vi "NanotecSMCPD.ProcPeriodic.vi"(0 "i ref in":refnum<vi>, 3 "ms timeout (10000)":i32=10000, 5 "error in (no error)":errorcluster) -> (14 "i ref out":refnum<vi>, 17 "timed out":bool, 19 "error out":errorcluster)   [LabVIEW 2014, in "NanotecSMCPD.lvlib"]
doc: "This method serves to periodically do things like reading values from the HW. Methods that should be executed periodically should be called from THIS method. Add code here."
uses:
  NanotecSMCPD.lvlib
  CSCore/CSSystem/CoreDefs/CoreDefs.error_type.ctl
  CSCore/CSSystem/CoreDefs/CoreDefs.error_severity.ctl
  CSCore/CSApplicationBaseClasses/MotorBase/MotorBase.statusType.ctl
  CSCore/CSApplicationBaseClasses/MotorBase/MotorBase.lvlib
  CSCore/CSSystem/CoreLib/CoreLib.lvlib
  CSlibraries/UtilityLib/UtilityLib.lvlib
  CSlibraries-extern/DimLVEvent/LVDimInterface/LVDimInterface.lvlib
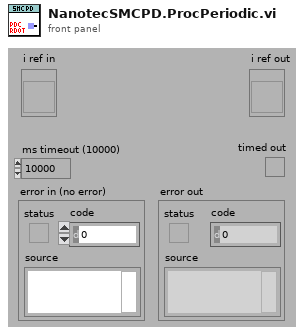
[diagram p1: front panel]
types:
  T1 = typedef "CoreDefs.error_severity.ctl" = enum16{"undefined", "information", "warning", "error", "fatal"}
  T2 = typedef "CoreDefs.error_type.ctl" = enum16{"no error", "can't load process", "can't unload process", "process does not exist", "can't install process", "can't remove process", "unknown function", "time out", "can't execute function", "duplicate queue name", "super not found", "caller queue invalid", "can't ping process", "unknown error", "VISA Error", "VISA timeout", "GPIB timeout", "GPIB error", "communication error", "data type mismatch", "can't read data from OPC server", "can't write data to OPC server", "OET error", "function not implemented", "process already exists", "invalid Shared Variable name", "error writing Shared Variable", "error reading Shared Variable", "invalid client name", "corrupt database", "unknown class", "call not authorized", "parameter out of range", "OET timeout: can't get data to modify", "invalid queue name", "requested operation incompatible with current state", "event undefined", "event disabled", "state undefined", "caller is not a friend", "EventBuilder: bad eventID", "EventBuilder: no DAQ devices", "a thread must not stop itself", "UNUSED ELEMENT4", "DiscArchiver: eventData incomplete", "DiscArchiver: eventData does not belong to run", "DiscArchiver: can't open file", "DiscArchiver: can't write to file", "DiscArchiver: available disc space low", "can't acquire semaphore", "error reading data from database", "notifier object is not existing", "can't register process", "can't unregister process", "illegal event type", "object disabled", "object already exists", "can't change state", "Instrument not found", "no connection to remote node", "invalid reference", "N/A", "UNUSED ELEMENT 1", "element not found", "illegal TCP/IP connection detected", "object does not exist", "invalid access ID", "unknown CS system", "invalid privilige", "unsupported data type", "unsupported server type", "IO server already exists", "Shared Variable already exists"}
  T3 = typedef "MotorBase.lvlib/MotorBase.statusType.ctl" = u32
  T4 = typedef "NanotecSMCPD.lvlib/NanotecSMCPD.i attribute.ctl" = cluster{"referencing":bool[], "stop":bool[], "AutoHalt ID":i32, "MethodQueue":refnum<queue>, "Referenced1Time?":bool[], "LastCommand ID":i32}
  T5 = cluster{"Method":enum16{"MoveRelative", "MoveAbsolute", "Stop"}, "Axis":i32, "Steps":dbl}
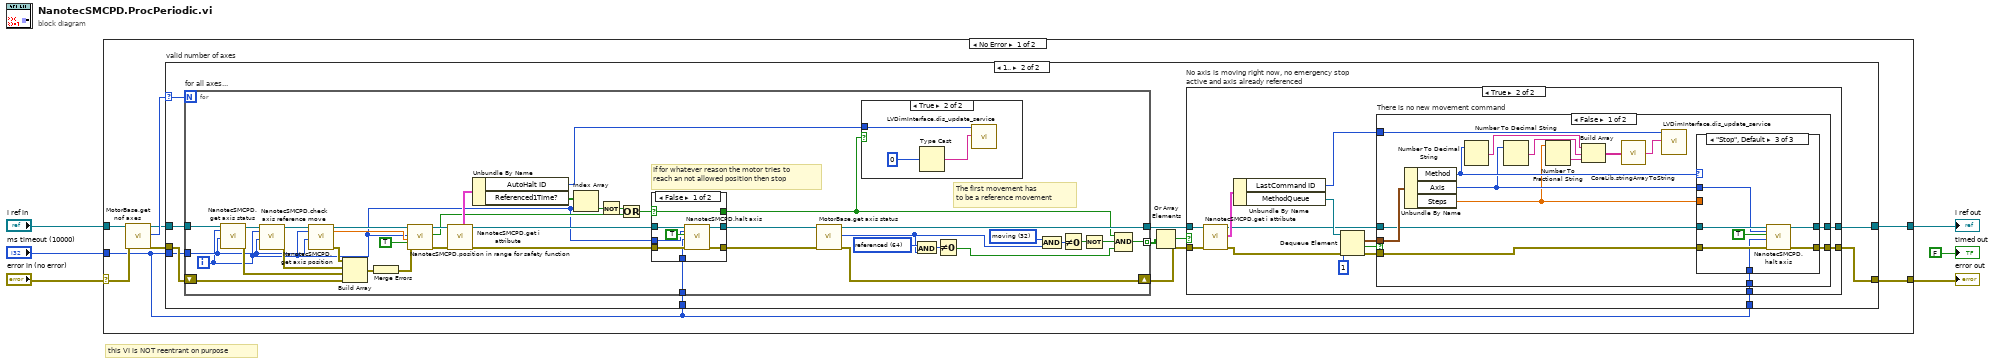
[diagram p0: block diagram]
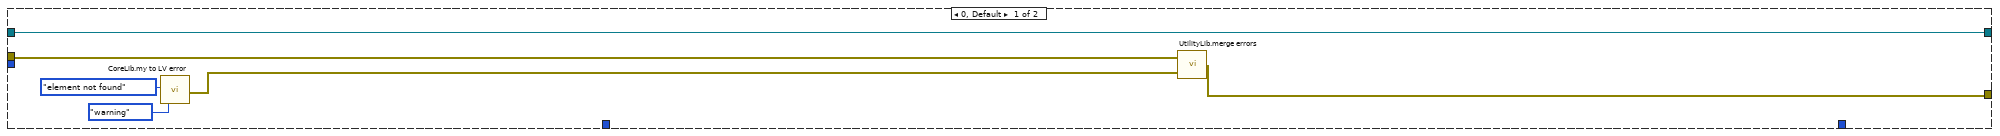
[diagram p2: hidden frame]
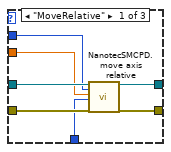
[diagram p4: hidden frame]
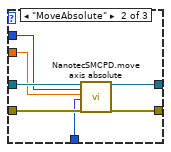
[diagram p5: hidden frame]
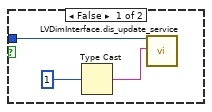
[diagram p7: hidden frame]
diagram:
  # "this VI is NOT reentrant on purpose"
  n1 = case shown="No Error" "error in (no error)" {
    selector: "error in (no error)" -> [w11 w144]
    tunnel: "i ref in" -> [w12 w145]
    tunnel: [w14 w145] -> w4
    tunnel: [w13 w144] -> w3
    tunnel: "ms timeout (10000)" -> [w7 _]
    frame No Error {
      n2 = call "MotorBase.get nof axes.vi"("i ref in"=w12, "error in (no error)"=w11) -> ("i ref out"=w9:refnum<vi>, "nOfAxis"=w10:i32, "error out"=w8:errorcluster)  [unwired: 15 in]
      n3 = case "valid number of axes" shown="1.." w10 {
        selector: w10 -> [_ w30]
        tunnel: [w20 w24] -> w14
        tunnel: w9 -> [w20 w32]
        tunnel: w8 -> [w17 w31]
        tunnel: [w15 w23] -> w13
        tunnel: w7 -> [_ w29]
        tunnel: w7 -> [_ w25]
        tunnel: w7 -> [_ w21]
        frame 0, Default {
          n4 = call "CoreLib.my to LV error.vi"("ErrorTypes"=CoreDefs.error_type."element not found", "severityLevel"=CoreDefs.error_severity."warning") -> ("myErrorCluster"=w16:errorcluster)  [unwired: 16 in, 1 out]
          n5 = call "UtilityLib.merge errors.vi"("error2 (no error)"=w16, "error1 (no error)"=w17) -> ("error out"=w15:errorcluster)
        }
        frame 1.. {
          n6 = for "for all axes..." {
            N: w30 -> [_]
            tunnel: w32 -> [w87]
            shift-right: [w121] -> w26
            shift-left: w31 -> [w125]
            tunnel: w29 -> [w89]
            tunnel: [w120] -> w27
            tunnel: [w98] -> w28 mode=indexing
            tunnel: w21 -> [w104]
            i -> [w88]
            w116 = T3 64 items=["motorEnabled"=1, "negativeLimitSwitchActive"=2, "positiveLimitSwitchActive"=4, "limitSwitchesEnabled"=8, "limitSwitchesAreNormallyClosed"=16, "moving"=32, "referenced"=64, "inPosition"=128, "reserved2"=256, "reserved3"=512, "reserved4"=1024, "reserved5"=2048, "error"=4096, "reserved6"=8192, "reserved7"=16384, "reserved8"=32768, "user defined1"=65536, "user defined2"=131072, "user defined3"=262144, "user defined4"=524288, "user defined5"=1048576, "user defined6"=2097152, "user defined7"=4194304, "user defined8"=8388608, "user defined9"=16777216, "user defined10"=33554432, "user defined11"=67108864, "user defined12"=134217728, "user defined13"=268435456, "user defined14"=536870912, "user defined15"=1073741824, "user defined16"=2147483648] ("status")
            w122 = T3 32 items=["motorEnabled"=1, "negativeLimitSwitchActive"=2, "positiveLimitSwitchActive"=4, "limitSwitchesEnabled"=8, "limitSwitchesAreNormallyClosed"=16, "moving"=32, "referenced"=64, "inPosition"=128, "reserved2"=256, "reserved3"=512, "reserved4"=1024, "reserved5"=2048, "error"=4096, "reserved6"=8192, "reserved7"=16384, "reserved8"=32768, "user defined1"=65536, "user defined2"=131072, "user defined3"=262144, "user defined4"=524288, "user defined5"=1048576, "user defined6"=2097152, "user defined7"=4194304, "user defined8"=8388608, "user defined9"=16777216, "user defined10"=33554432, "user defined11"=67108864, "user defined12"=134217728, "user defined13"=268435456, "user defined14"=536870912, "user defined15"=1073741824, "user defined16"=2147483648] ("status")
            # "The first movement has\nto be a reference movement"
            # "If for whatever reason the motor tries to\nreach an not allowed position then stop"
            n7 = call "NanotecSMCPD.get axis status.vi"("i ref in"=w87, "axis"=w88, "ms timeout (10000)"=w89) -> ("i ref out"=w126:refnum<vi>, "error out"=w92:errorcluster)  [unwired: 12 in, 3 out]
            n8 = call "NanotecSMCPD.check axis reference move.vi"("i ref in"=w126, "axis"=w88, "ms timeout (10000)"=w89) -> ("i ref out"=w95:refnum<vi>, "error out"=w91:errorcluster)  [unwired: 14 in, 1 out]
            n9 = call "NanotecSMCPD.get axis position.vi"("i ref in"=w95, "axis"=w88, "ms timeout (10000)"=w89) -> ("i ref out"=w94:refnum<vi>, "position [unit]"=w93:dbl, "error out"=w90:errorcluster)  [unwired: 13 in, 1 out]
            n10 = Build Array(w90, w91, w92, w125) -> (w124:errorcluster[])
            n11 = Merge Errors(w124) -> (w119:errorcluster)
            n12 = call "NanotecSMCPD.position in range for safety function.vi"("i ref in"=w94, "axisIndex"=w88, "reqPosition"=w93, "absolute"=TRUE, "error in (no error)"=w119) -> ("i ref out"=w114:refnum<vi>, "in range"=w110:bool, "error out"=w113:errorcluster)  [unwired: 12 in]
            n13 = call "NanotecSMCPD.get i attribute.vi"("i ref in"=w114, "error in (no error)"=w113) -> ("i ref out"=w108:refnum<vi>, "i attribute"=w112:T4, "error out"=w107:errorcluster)  [unwired: 15 in]
            n14 = Unbundle By Name(w112) -> ("AutoHalt ID"=w96:i32, "Referenced1Time?"=w111:bool[])
            n15 = Index Array(array=w111, index=w88) -> (element=w103:bool)
            n16 = Not(x=w103) -> (.not. x?=w102:bool)
            n17 = Or(x=w102, y=w110) -> (x .or. y?=w109:bool)
            n18 = case shown="False" w109 {
              selector: w109 -> [w133 w141]
              tunnel: w108 -> [w139 w143]
              tunnel: w107 -> [w138 w142]
              tunnel: [w137 w143] -> w106
              tunnel: [w136 w142] -> w105
              tunnel: w88 -> [w135 _]
              tunnel: w104 -> [w134 _]
              tunnel: [w133 w141] -> w97
              frame False {
                n19 = call "NanotecSMCPD.halt axis.vi"("i ref in"=w139, "axis"=w135, "ManuelStop"=TRUE, "ms timeout (10000)"=w134, "error in (no error)"=w138) -> ("i ref out"=w137:refnum<vi>, "error out"=w136:errorcluster)  [unwired: 12 in, 1 out]
              }
              frame True {
              }
            }
            n20 = call "MotorBase.get axis status.vi"("i ref in"=w106, "error in (no error)"=w105) -> ("i ref out"=w120:refnum<vi>, "status"=w115:T3, "error out"=w121:errorcluster)  [unwired: 15 in]
            n21 = case shown="True" w97 {
              tunnel: w96 -> [w127 w130]
              frame False {
                n22 = Type Cast(x=1) -> (*(type *) &x=w128:string)  [unwired: 1 in]
                n23 = call "LVDimInterface.dis_update_service.vi"("my_serviceID"=w127, "data"=w128) -> ()  [unwired: 15 in, 3 out]
              }
              frame True {
                n24 = Type Cast(x=0) -> (*(type *) &x=w131:string)  [unwired: 1 in]
                n25 = call "LVDimInterface.dis_update_service.vi"("my_serviceID"=w130, "data"=w131) -> ()  [unwired: 15 in, 3 out]
              }
            }
            n26 = And(x=w116, y=w115) -> (x .and. y?=w117:T3)
            n27 = Not Equal To 0?(x=w117) -> (x != 0?=w99:bool)
            n28 = And(x=w122, y=w115) -> (x .and. y?=w123:T3)
            n29 = Not Equal To 0?(x=w123) -> (x != 0?=w101:bool)
            n30 = Not(x=w101) -> (.not. x?=w100:bool)
            n31 = Compound Arithmetic op=AND(w97, w100, w99) -> (w98:bool)
          }
          n32 = Or Array Elements(Boolean array=w28) -> (logical OR=w22:bool)
          n33 = case "No axis is moving right now, no emergency stop active and axis already referenced" shown="True" w22 {
            tunnel: w27 -> [w34 w46]
            tunnel: w26 -> [w33 w45]
            tunnel: w25 -> [_ w38]
            tunnel: [w34 w37] -> w24
            tunnel: [w33 w36] -> w23
            frame False {
            }
            frame True {
              n34 = call "NanotecSMCPD.get i attribute.vi"("i ref in"=w46, "error in (no error)"=w45) -> ("i ref out"=w39:refnum<vi>, "i attribute"=w47:T4, "error out"=w44:errorcluster)  [unwired: 15 in]
              n35 = Unbundle By Name(w47) -> ("LastCommand ID"=w35:i32, "MethodQueue"=w48:refnum<queue>)
              n36 = Dequeue Element(queue=w48, timeout in ms (-1)=1, error in (no error)=w44) -> (element=w41:T5, timed out?=w42:bool, error out=w40:errorcluster)  [unwired: 1 out]
              n37 = case "There is no new movement command" shown="False" w42 {
                tunnel: w41 -> [w63 _]
                tunnel: w40 -> [w61 w85]
                tunnel: w39 -> [w62 w86]
                tunnel: w38 -> [w60 _]
                tunnel: [w59 w86] -> w37
                tunnel: [w58 w85] -> w36
                tunnel: w35 -> [w57 _]
                frame False {
                  n38 = Unbundle By Name(w63) -> ("Method"=w56:enum16{"MoveRelative", "MoveAbsolute", "Stop"}, "Axis"=w55:i32, "Steps"=w54:dbl)
                  n39 = Number To Decimal String(number=w56) -> (decimal integer string=w53:string)  [unwired: 1 in]
                  n40 = Number To Decimal String(number=w55) -> (decimal integer string=w52:string)  [unwired: 1 in]
                  n41 = Number To Fractional String(number=w54) -> (F-format string=w51:string)  [unwired: 3 in]
                  n42 = Build Array(w53, w52, w51) -> (w50:string[])
                  n43 = call "CoreLib.stringArrayToString.vi"("Array"=w50) -> ("String"=w49:string)
                  n44 = call "LVDimInterface.dis_update_service.vi"("my_serviceID"=w57, "data"=w49) -> ()  [unwired: 15 in, 3 out]
                  n45 = case shown="\"Stop\", Default" w56 {
                    tunnel: w62 -> [w70 w77 w84]
                    tunnel: w61 -> [w69 w76 w83]
                    tunnel: w54 -> [w65 w75 _]
                    tunnel: w55 -> [w64 w74 w79]
                    tunnel: w60 -> [w66 w73 w80]
                    tunnel: [w67 w72 w82] -> w59
                    tunnel: [w68 w71 w81] -> w58
                    frame "MoveRelative" {
                      n46 = call "NanotecSMCPD.move axis relative.vi"("i ref in"=w70, "axis"=w64, "relPosition"=w65, "ms timeout (10000)"=w66, "error in (no error)"=w69) -> ("i ref out"=w67:refnum<vi>, "error out"=w68:errorcluster)  [unwired: 12 in, 1 out]
                    }
                    frame "MoveAbsolute" {
                      n47 = call "NanotecSMCPD.move axis absolute.vi"("i ref in"=w77, "axis"=w74, "absPosition [unit]"=w75, "ms timeout (10000)"=w73, "error in (no error)"=w76) -> ("i ref out"=w72:refnum<vi>, "error out"=w71:errorcluster)  [unwired: 12 in, 1 out]
                    }
                    frame "Stop", Default {
                      n48 = call "NanotecSMCPD.halt axis.vi"("i ref in"=w84, "axis"=w79, "ManuelStop"=TRUE, "ms timeout (10000)"=w80, "error in (no error)"=w83) -> ("i ref out"=w82:refnum<vi>, "error out"=w81:errorcluster)  [unwired: 12 in, 1 out]
                    }
                  }
                }
                frame True {
                }
              }
            }
          }
        }
      }
    }
    frame Error {
    }
  }
  "error out" <- w3
  "i ref out" <- w4
  "timed out" <- FALSE ("timed out")
